vi "Eltochpribor RRG.vi"() -> ()   [LabVIEW 2015]
uses:
  Eltochpribor RRG.lvclass
panel:
  in  "set zero":bool
  in  "flow rate, %":dbl
  out "measured flow rate, %":dbl
  in  "valve mode":u8(ring) items=["auto", "open", "closed"]
  in  "timeout, ms":u32=300
  in  "address":u8=1
  in  "baud rate":u32=19200
  in  "port":refnum<visa-resource-name>
  out "RRG":refnum<class "Eltochpribor RRG.lvclass">
  out "error":errorcluster
  in  "stop":bool
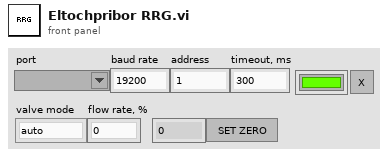
[diagram p1: front panel]
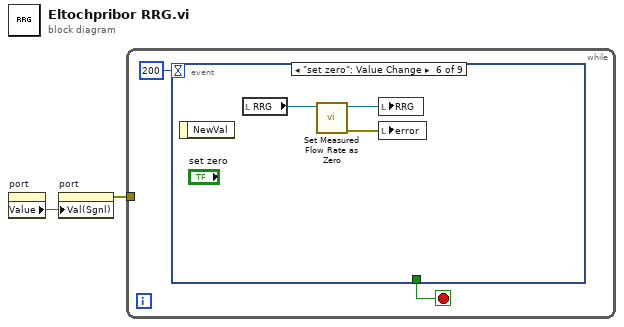
[diagram p0: block diagram]
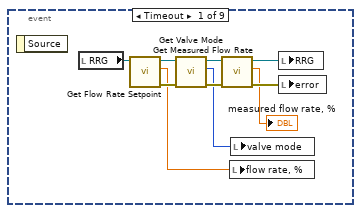
[diagram p2: hidden frame]
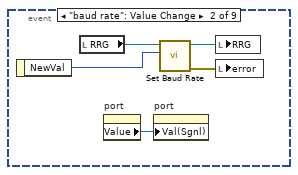
[diagram p3: hidden frame]
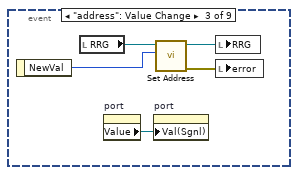
[diagram p4: hidden frame]
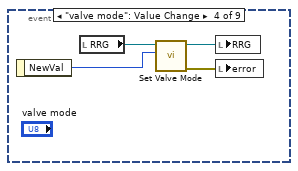
[diagram p5: hidden frame]
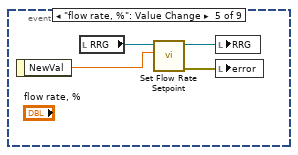
[diagram p6: hidden frame]
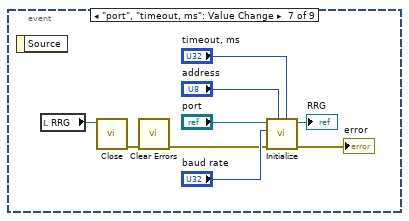
[diagram p7: hidden frame]
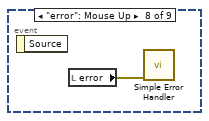
[diagram p8: hidden frame]
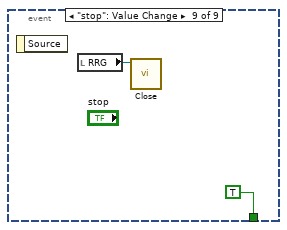
[diagram p9: hidden frame]
diagram:
  n1 = property on="port" class="VISAName"() -> ("Value"=w1:refnum<visa-resource-name>)  [unwired: 2 in, 2 out]
  n2 = property on="port" class="VISAName"("Val(Sgnl)"=w1) -> (error out=w2:errorcluster)  [unwired: 2 in, 1 out]
  n3 = while {
    tunnel: w2 -> [_]
    stop <- w3 stop-if-true
    n4 = event shown="[5] \"set zero\": Value Change" {
      selector: _ -> [_ _ _ _ _ _ _ _ _]
      dyn-events: _ -> [_ _ _ _ _ _ _ _ _]
      timeout: 200 -> [_ _ _ _ _ _ _ _ _]
      tunnel: [_ _ _ _ _ _ _ _ TRUE ("stop")] -> w3
      event Timeout {
        n5 = event-data() -> ()  [unwired: 1 in, 1 out]
        n6 = local read "RRG"() -> (w8:refnum<class "Eltochpribor RRG.lvclass">)
        n7 = call "Get Flow Rate Setpoint.vi"("RRG in"=w8) -> ("error out"=w14:errorcluster, "flow rate setpoint, %"=w5:dbl, "RRG out"=w10:refnum<class "Eltochpribor RRG.lvclass">)  [unwired: 8 in]
        n8 = call "Get Valve Mode.vi"("error in (no error)"=w14, "RRG in"=w10) -> ("error out"=w13:errorcluster, "valve mode"=w7:u8, "RRG out"=w11:refnum<class "Eltochpribor RRG.lvclass">)  [unwired: 7 in]
        n9 = call "Get Measured Flow Rate.vi"("error in (no error)"=w13, "RRG in"=w11) -> ("error out"=w9:errorcluster, "measured flow rate, %"=→"measured flow rate, %":dbl, "RRG out"=w12:refnum<class "Eltochpribor RRG.lvclass">)  [unwired: 7 in]
        n10 = local write "flow rate, %"(w5) -> ()
        n11 = local write "valve mode"(w7) -> ()
        n12 = local write "RRG"(w12) -> ()
        n13 = local write "error"(w9) -> ()
      }
      event "baud rate": Value Change {
        n14 = event-data() -> ("NewVal"=w15:u32)  [unwired: 1 in]
        n15 = local read "RRG"() -> (w18:refnum<class "Eltochpribor RRG.lvclass">)
        n16 = property on="port" class="VISAName"() -> ("Value"=w19:refnum<visa-resource-name>)  [unwired: 2 in, 2 out]
        n17 = property on="port" class="VISAName"("Val(Sgnl)"=w19) -> ()  [unwired: 2 in, 2 out]
        n18 = call "Set Baud Rate.vi"("baud rate"=w15, "RRG in"=w18) -> ("error out"=w16:errorcluster, "RRG out"=w17:refnum<class "Eltochpribor RRG.lvclass">)  [unwired: 8 in]
        n19 = local write "RRG"(w17) -> ()
        n20 = local write "error"(w16) -> ()
      }
      event "address": Value Change {
        n21 = event-data() -> ("NewVal"=w20:u8)  [unwired: 1 in]
        n22 = local read "RRG"() -> (w21:refnum<class "Eltochpribor RRG.lvclass">)
        n23 = property on="port" class="VISAName"() -> ("Value"=w24:refnum<visa-resource-name>)  [unwired: 2 in, 2 out]
        n24 = property on="port" class="VISAName"("Val(Sgnl)"=w24) -> ()  [unwired: 2 in, 2 out]
        n25 = call "Set Address.vi"("address"=w20, "RRG in"=w21) -> ("error out"=w22:errorcluster, "RRG out"=w23:refnum<class "Eltochpribor RRG.lvclass">)  [unwired: 8 in]
        n26 = local write "RRG"(w23) -> ()
        n27 = local write "error"(w22) -> ()
      }
      event "valve mode": Value Change {
        n28 = event-data() -> ("NewVal"=w25:u8)  [unwired: 1 in]
        n29 = local read "RRG"() -> (w28:refnum<class "Eltochpribor RRG.lvclass">)
        n30 = call "Set Valve Mode.vi"("valve mode"=w25, "RRG in"=w28) -> ("error out"=w27:errorcluster, "RRG out"=w26:refnum<class "Eltochpribor RRG.lvclass">)  [unwired: 8 in]
        n31 = local write "RRG"(w26) -> ()
        n32 = local write "error"(w27) -> ()
      }
      event "flow rate, %": Value Change {
        n33 = event-data() -> ("NewVal"=w29:dbl)  [unwired: 1 in]
        n34 = local read "RRG"() -> (w30:refnum<class "Eltochpribor RRG.lvclass">)
        n35 = call "Set Flow Rate Setpoint.vi"("flow rate setpoint, %"=w29, "RRG in"=w30) -> ("error out"=w31:errorcluster, "RRG out"=w32:refnum<class "Eltochpribor RRG.lvclass">)  [unwired: 8 in]
        n36 = local write "RRG"(w32) -> ()
        n37 = local write "error"(w31) -> ()
      }
      event "set zero": Value Change {
        n38 = event-data() -> ()  [unwired: 1 in, 1 out]
        n39 = local read "RRG"() -> (w34:refnum<class "Eltochpribor RRG.lvclass">)
        n40 = call "Set Measured Flow Rate as Zero.vi"("RRG in"=w34) -> ("error out"=w35:errorcluster, "RRG out"=w33:refnum<class "Eltochpribor RRG.lvclass">)  [unwired: 9 in]
        n41 = local write "RRG"(w33) -> ()
        n42 = local write "error"(w35) -> ()
      }
      event "port", "timeout, ms": Value Change {
        n43 = event-data() -> ()  [unwired: 1 in, 1 out]
        n44 = local read "RRG"() -> (w38:refnum<class "Eltochpribor RRG.lvclass">)
        n45 = call-dynamic "Close.vi"("RRG in"=w38) -> ("error out"=w37:errorcluster)  [unwired: 10 in]
        n46 = call <vilib>:"Clear Errors.vi"("error in (no error)"=w37) -> ("error out"=w36:errorcluster)  [unwired: 5 in, 1 out]
        n47 = call "Initialize.vi"("timeout, ms (300)"="timeout, ms", "address (1)"="address", "error in (no error)"=w36, "baud rate (19200)"="baud rate", "port"="port") -> ("error out"=→"error":errorcluster, "RRG out"=→"RRG":refnum<class "Eltochpribor RRG.lvclass">)  [unwired: 5 in]
      }
      event "error": Mouse Up {
        n48 = event-data() -> ()  [unwired: 1 in, 1 out]
        n49 = local read "error"() -> (w45:errorcluster)
        n50 = call <vilib>:"Simple Error Handler.vi"("error in (no error)"=w45) -> ()  [unwired: 4 in, 5 out]
      }
      event "stop": Value Change {
        n51 = event-data() -> ()  [unwired: 1 in, 1 out]
        n52 = local read "RRG"() -> (w47:refnum<class "Eltochpribor RRG.lvclass">)
        n53 = call-dynamic "Close.vi"("RRG in"=w47) -> ()  [unwired: 10 in, 1 out]
      }
    }
  }
